vi "Table, Set Column Color.vi"(4 "Enable":bool=TRUE, 5 "BGColor Default":u32(colorbox)=16777215, 6 "BGColor Enabled":u32(colorbox)=16448250, 7 "error in":errorcluster, 9 "col (0)":i32, 10 "Tbl Refnum":refnum<vi>) -> (0 "error out":errorcluster, 3 "Tbl Refnum out":refnum<vi>)   [LabVIEW 2010]
doc: "Sets the background color attribute for each cell in a table column."
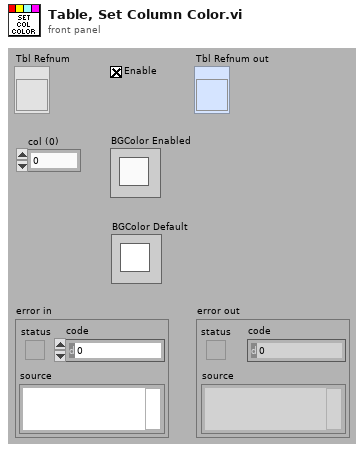
[diagram p1: front panel]
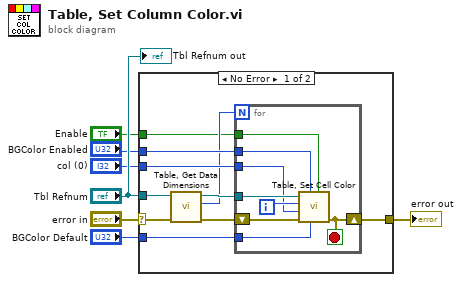
[diagram p0: block diagram]
diagram:
  n1 = case shown="No Error" "error in" {
    selector: "error in" -> [w14 w26]
    tunnel: "Tbl Refnum" -> [w16 _]
    tunnel: [w17 w26] -> w6
    tunnel: "col (0)" -> [w12 _]
    tunnel: "BGColor Enabled" -> [w11 _]
    tunnel: "BGColor Default" -> [w9 _]
    tunnel: "Enable" -> [w8 _]
    frame No Error {
      n2 = call "Table, Get Data Dimensions.vi"("error in"=w14, "Tbl Refnum"=w16) -> ("error out"=w13:errorcluster, "row_n"=w10:i32, "Tbl Refnum out"=w15:refnum<vi>)  [unwired: 6 in, 1 out]
      n3 = for {
        N: w10 -> [_]
        shift-right: [w18] -> w17
        shift-left: w13 -> [w25]
        tunnel: w15 -> [w24]
        tunnel: w12 -> [w22]
        tunnel: w11 -> [w21]
        tunnel: w9 -> [w20]
        tunnel: w8 -> [w19]
        i -> [w23]
        stop <- w18 stop-if-true
        n4 = call "Table, Set Cell Color.vi"("Enable (T)"=w19, "BGColor Default"=w20, "BGColor Enabled"=w21, "error in"=w25, "col (0)"=w22, "row (0)"=w23, "Tbl Refnum"=w24) -> ("error out"=w18:errorcluster)  [unwired: 3 out]
      }
    }
    frame Error {
    }
  }
  "error out" <- w6
  "Tbl Refnum out" <- "Tbl Refnum"
